vi "UnLoadScanPanel.vi"(8 "error in (no error)":errorcluster caption="entrée d'erreur (pas d'erreur)", 9 "ScanIndex":i32[][](array[numeric]), 10 "SubPanRef":refnum<vi>, 11 "LoadedInst":refnum<class "BaseDevice.lvclass">[](array[class])) -> (0 "sortie d'erreur":errorcluster, 3 "LoadedInst Out":refnum<class "BaseDevice.lvclass">[](array[class]) caption="LoadedInst")   [LabVIEW 2019, in "BaseDevice.lvclass"]
uses:
  BaseDevice.lvclass
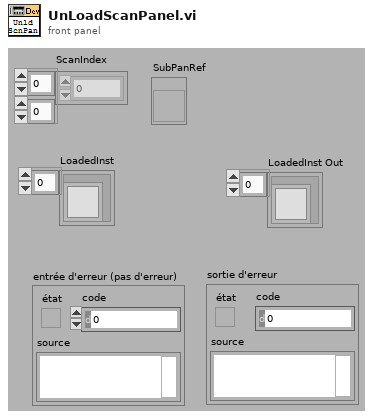
[diagram p1: front panel]
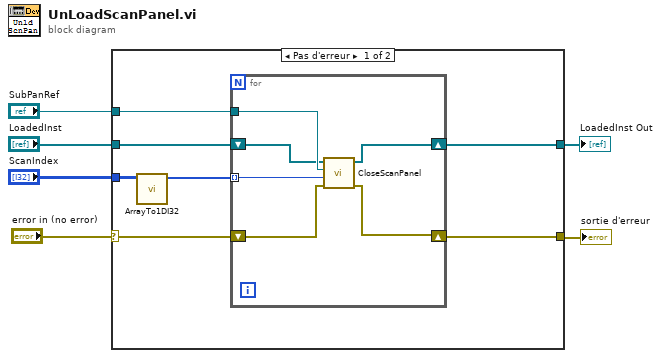
[diagram p0: block diagram]
diagram:
  n1 = case shown="Pas d'erreur" "error in (no error)" {
    selector: "error in (no error)" -> [w11 w20]
    tunnel: [w10 w20] -> w5
    tunnel: [w12 w21] -> w3
    tunnel: "LoadedInst" -> [w13 w21]
    tunnel: "ScanIndex" -> [w8 _]
    tunnel: "SubPanRef" -> [w9 _]
    frame No Error {
      n2 = call <userlib>:"ArrayTo1DI32.vi"("tableau"=w8) -> ("Array Out"=w7:i32[])  [unwired: 8 in, 2 out]
      n3 = for {
        shift-right: [w15] -> w12
        shift-left: w13 -> [w16]
        tunnel: w7 -> [w14] mode=indexing
        shift-right: [w18] -> w10
        shift-left: w11 -> [w19]
        tunnel: w9 -> [w17]
        n4 = call "CloseScanPanel.vi"("error in (no error)"=w19, "Index"=w14, "SubPanRef"=w17, "LoadedInst"=w16) -> ("sortie d'erreur"=w18:errorcluster, "LoadedInst Out"=w15:refnum<class "BaseDevice.lvclass">[])  [unwired: 6 in]
      }
    }
    frame Error {
    }
  }
  "sortie d'erreur" <- w5
  "LoadedInst Out" <- w3
